vi "Vision Demo.vi"() -> ()   [LabVIEW 2015]
panel:
  out "Vision Data":T1
  in  "stop":bool
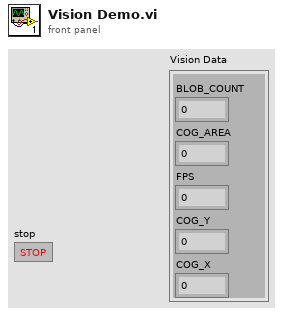
[diagram p1: front panel]
types:
  T1 = cluster{"COG_X":dbl, "COG_Y":dbl, "FPS":dbl, "COG_AREA":dbl, "BLOB_COUNT":dbl}
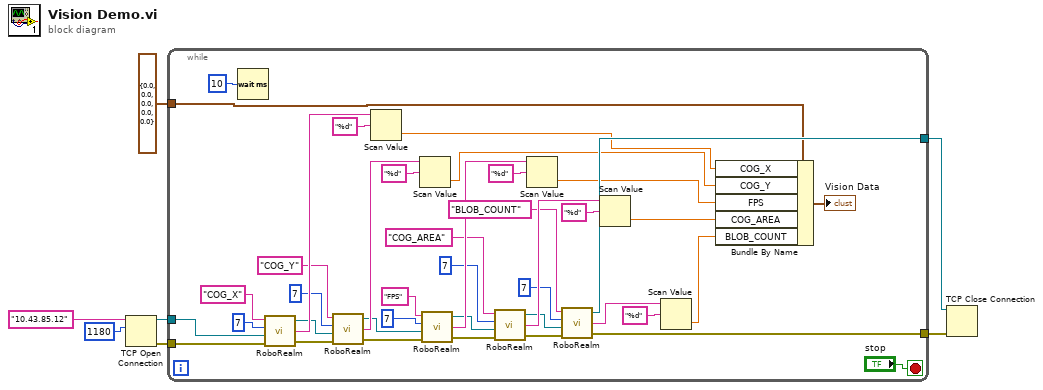
[diagram p0: block diagram]
diagram:
  n1 = TCP Open Connection(address="10.43.85.12", remote port or service name=u16 1180) -> (connection ID=w7:refnum<k5>, error out=w3:errorcluster)  [unwired: 3 in]
  n2 = while {
    tunnel: w7 -> [w43]
    tunnel: [w21] -> w4
    tunnel: w3 -> [w20]
    tunnel: [w15] -> w2
    tunnel: T1 {"COG_X"=0.0, "COG_Y"=0.0, "FPS"=0.0, "COG_AREA"=0.0, "BLOB_COUNT"=0.0} ("Vision Data") -> [w8]
    stop <- "stop" stop-if-true
    n3 = Wait (ms)(milliseconds to wait=u32 10) -> ()  [unwired: 1 out]
    n4 = call "RoboRealm.vi"("error in (no error)"=w20, "connection ID IN"=w43, "Max Variable Length"=7, "Variable Name"="COG_X") -> ("error out"=w19:errorcluster, "Variable Value"=w45:string, "connection ID out"=w32:refnum<k5>)
    n5 = call "RoboRealm.vi"("error in (no error)"=w19, "connection ID IN"=w32, "Max Variable Length"=7, "Variable Name"="COG_Y") -> ("error out"=w18:errorcluster, "Variable Value"=w40:string, "connection ID out"=w33:refnum<k5>)
    n6 = Scan Value(string=w45, format string="%d") -> (value=w14:dbl)  [unwired: 1 in, 1 out]
    n7 = Scan Value(string=w40, format string="%d") -> (value=w13:dbl)  [unwired: 1 in, 1 out]
    n8 = call "RoboRealm.vi"("error in (no error)"=w18, "connection ID IN"=w33, "Max Variable Length"=7, "Variable Name"="FPS") -> ("error out"=w17:errorcluster, "Variable Value"=w35:string, "connection ID out"=w23:refnum<k5>)
    n9 = call "RoboRealm.vi"("error in (no error)"=w17, "connection ID IN"=w23, "Max Variable Length"=7, "Variable Name"="COG_AREA") -> ("error out"=w16:errorcluster, "Variable Value"=w30:string, "connection ID out"=w22:refnum<k5>)
    n10 = Scan Value(string=w35, format string="%d") -> (value=w12:dbl)  [unwired: 1 in, 1 out]
    n11 = call "RoboRealm.vi"("error in (no error)"=w16, "connection ID IN"=w22, "Max Variable Length"=7, "Variable Name"="BLOB_COUNT") -> ("error out"=w15:errorcluster, "Variable Value"=w25:string, "connection ID out"=w21:refnum<k5>)
    n12 = Scan Value(string=w30, format string="%d") -> (value=w11:dbl)  [unwired: 1 in, 1 out]
    n13 = Scan Value(string=w25, format string="%d") -> (value=w10:dbl)  [unwired: 1 in, 1 out]
    n14 = Bundle By Name(cluster=w8, "COG_X"=w14, "COG_Y"=w13, "FPS"=w12, "COG_AREA"=w11, "BLOB_COUNT"=w10) -> (→"Vision Data":T1)
  }
  n15 = TCP Close Connection(connection ID=w4, error in (no error)=w2) -> ()  [unwired: 1 in, 2 out]
